vi "LED-Matrix-poc.vi"() -> ()   [LabVIEW 2026]
uses:
  CTI-Grove/Examples/Sourcecode/cti-drivers-lv-visa-simple/Examples/Driver/CTIPicoVISA.lvlib
panel:
  out "Identity":T1
  out "Numeric":i32
  out "error out":errorcluster
  in  "stop":bool
  in  "VISA resource name in":refnum<visa-resource-name>="ASRL1::INSTR"
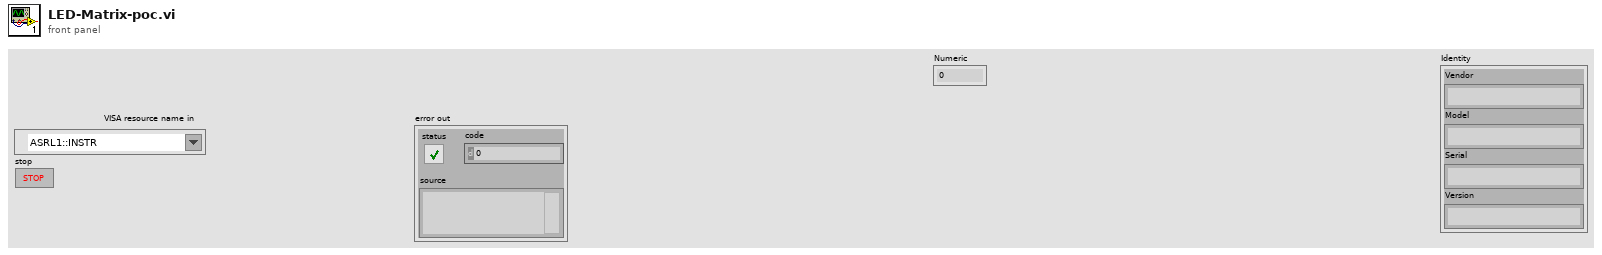
[diagram p1: front panel]
types:
  T1 = cluster{"Vendor":string, "Model":string, "Serial":string, "Version":string}
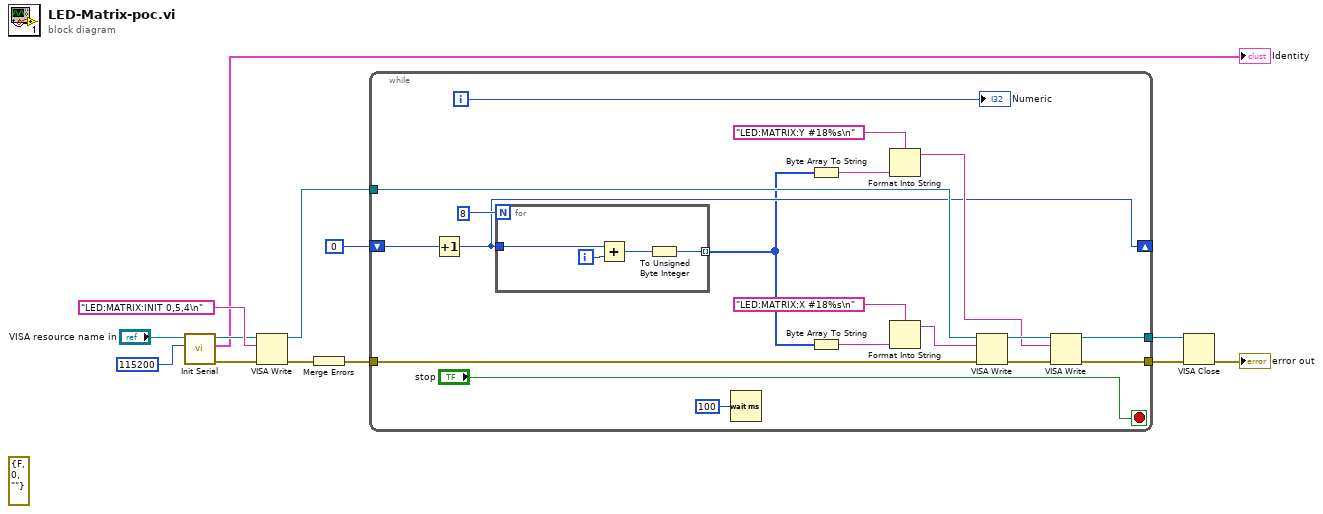
[diagram p0: block diagram]
diagram:
  (unwired) errorcluster {"status"=FALSE, "code"=0, "source"=""} ("error in (no error)")
  n1 = call "Init Serial.vi"("Baud (115200)"=u32 115200, "VISA resource name in"="VISA resource name in") -> ("error out"=w3:errorcluster, "Identity"=→"Identity":T1, "VISA resource name Out"=w4:refnum<visa-resource-name>)  [unwired: 7 in]
  n2 = VISA Write(VISA resource name=w4, write buffer="LED:MATRIX:INIT 0,5,4\n", error in (no error)=w3) -> (VISA resource name out=w12:refnum<visa-resource-name>, error out=w11:errorcluster)  [unwired: 1 out]
  n3 = Merge Errors(w11) -> (w10:errorcluster)
  n4 = while {
    tunnel: w12 -> [w32]
    tunnel: w10 -> [w31]
    tunnel: [w24] -> w9
    tunnel: [w26] -> w8
    shift-right: [w15] -> _
    shift-left: u8 0 -> [w17]
    i -> [w27]
    stop <- "stop" stop-if-true
    n5 = Increment(x=w17) -> (x+1=w15:u8)
    n6 = for {
      N: 8 -> [_]
      tunnel: w15 -> [w36]
      tunnel: [w33] -> w14 mode=indexing
      i -> [w35]
      n7 = Add(x=w36, y=w35) -> (x+y=w34:i32)
      n8 = To Unsigned Byte Integer(number=w34) -> (unsigned 8bit integer=w33:u8)
    }
    n9 = Wait (ms)(milliseconds to wait=u32 100) -> ()  [unwired: 1 out]
    n10 = Byte Array To String(unsigned byte array=w14) -> (string=w22:string)
    n11 = Byte Array To String(unsigned byte array=w14) -> (string=w20:string)
    n12 = Format Into String(format string="LED:MATRIX:Y #18%s\n" ("concatenated string"), w22) -> (resulting string=w21:string)  [unwired: 2 in, 1 out]
    n13 = Format Into String(format string="LED:MATRIX:X #18%s\n" ("concatenated string"), w20) -> (resulting string=w18:string)  [unwired: 2 in, 1 out]
    n14 = VISA Write(VISA resource name=w32, write buffer=w18, error in (no error)=w31) -> (VISA resource name out=w25:refnum<visa-resource-name>, error out=w28:errorcluster)  [unwired: 1 out]
    n15 = VISA Write(VISA resource name=w25, write buffer=w21, error in (no error)=w28) -> (VISA resource name out=w24:refnum<visa-resource-name>, error out=w26:errorcluster)  [unwired: 1 out]
    "Numeric" <- w27
  }
  n16 = VISA Close(VISA resource name=w9, error in (no error)=w8) -> (error out=→"error out":errorcluster)
